vi "Entry.vi"(8 "error in (no error)":errorcluster, 11 "Running in":refnum<class "Voice.lvclass">) -> (0 "error out":errorcluster, 3 "Running out":refnum<class "Voice.lvclass">)   [LabVIEW 2014, in "Voice.lvclass"]
doc: "This override sends a Start Acquisition message to the Process Actor. It also sends a Log Event message to the UI, with the string \"Entering Running State\" as its payload."
uses:
  Voice.lvclass
  Process State/CoordinatorState.lvclass
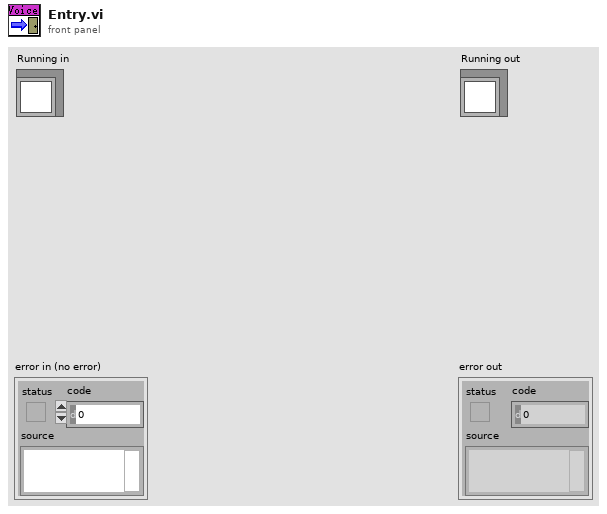
[diagram p1: front panel]
types:
  T1 = enum32{"Joy", "Map", "Voice", "Input", "Undefined"}
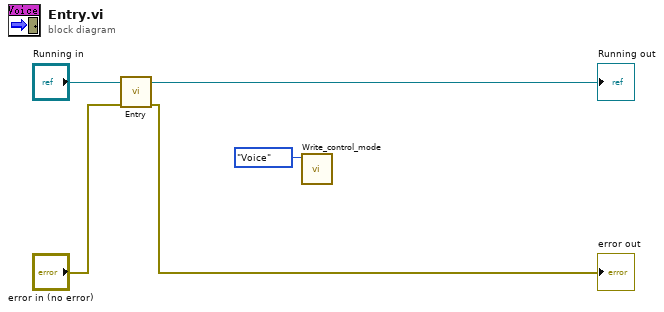
[diagram p0: block diagram]
diagram:
  n1 = call-parent "Entry.vi"("error in (no error)"="error in (no error)", "New State"="Running in") -> ("error out"=→"error out":errorcluster, "State out"=→"Running out":refnum<class "Voice.lvclass">)  [unwired: 8 in]
  n2 = call "Write_control_mode.vi"("Control_Mode"=T1."Voice") -> ()  [unwired: 11 in]
